vi "TSCAN_CANFD_Fold.vi"(10 "CANFD_Buffer输入":T1(array[cluster]), 11 "Fold Data":bool) -> (2 "CANFD_Buffer输出":T1(array[cluster]))   [LabVIEW 2014]
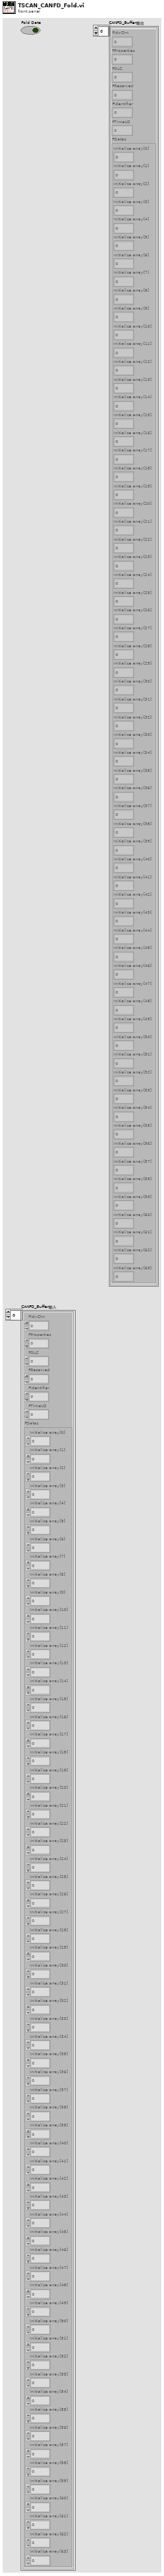
[diagram p1: front panel]
types:
  T1 = cluster{"FIdxChn":u8, "FProperties":u8, "FDLC":u8, "FReserved":u8, "FIdentifier":i32, "FTimeUS":u64, "FDatas":cluster{"Initialize array[0]":u8, "Initialize array[1]":u8, "Initialize array[2]":u8, "Initialize array[3]":u8, "Initialize array[4]":u8, "Initialize array[5]":u8, "Initialize array[6]":u8, "Initialize array[7]":u8, "Initialize array[8]":u8, "Initialize array[9]":u8, "Initialize array[10]":u8, "Initialize array[11]":u8, "Initialize array[12]":u8, "Initialize array[13]":u8, "Initialize array[14]":u8, "Initialize array[15]":u8, "Initialize array[16]":u8, "Initialize array[17]":u8, "Initialize array[18]":u8, "Initialize array[19]":u8, "Initialize array[20]":u8, "Initialize array[21]":u8, "Initialize array[22]":u8, "Initialize array[23]":u8, "Initialize array[24]":u8, "Initialize array[25]":u8, "Initialize array[26]":u8, "Initialize array[27]":u8, "Initialize array[28]":u8, "Initialize array[29]":u8, "Initialize array[30]":u8, "Initialize array[31]":u8, "Initialize array[32]":u8, "Initialize array[33]":u8, "Initialize array[34]":u8, "Initialize array[35]":u8, "Initialize array[36]":u8, "Initialize array[37]":u8, "Initialize array[38]":u8, "Initialize array[39]":u8, "Initialize array[40]":u8, "Initialize array[41]":u8, "Initialize array[42]":u8, "Initialize array[43]":u8, "Initialize array[44]":u8, "Initialize array[45]":u8, "Initialize array[46]":u8, "Initialize array[47]":u8, "Initialize array[48]":u8, "Initialize array[49]":u8, "Initialize array[50]":u8, "Initialize array[51]":u8, "Initialize array[52]":u8, "Initialize array[53]":u8, "Initialize array[54]":u8, "Initialize array[55]":u8, "Initialize array[56]":u8, "Initialize array[57]":u8, "Initialize array[58]":u8, "Initialize array[59]":u8, "Initialize array[60]":u8, "Initialize array[61]":u8, "Initialize array[62]":u8, "Initialize array[63]":u8}}[]
  T2 = cluster{"FIdxChn":u8, "FProperties":u8, "FDLC":u8, "FReserved":u8, "FIdentifier":i32, "FTimeUS":u64, "FDatas":cluster{"Initialize array[0]":u8, "Initialize array[1]":u8, "Initialize array[2]":u8, "Initialize array[3]":u8, "Initialize array[4]":u8, "Initialize array[5]":u8, "Initialize array[6]":u8, "Initialize array[7]":u8, "Initialize array[8]":u8, "Initialize array[9]":u8, "Initialize array[10]":u8, "Initialize array[11]":u8, "Initialize array[12]":u8, "Initialize array[13]":u8, "Initialize array[14]":u8, "Initialize array[15]":u8, "Initialize array[16]":u8, "Initialize array[17]":u8, "Initialize array[18]":u8, "Initialize array[19]":u8, "Initialize array[20]":u8, "Initialize array[21]":u8, "Initialize array[22]":u8, "Initialize array[23]":u8, "Initialize array[24]":u8, "Initialize array[25]":u8, "Initialize array[26]":u8, "Initialize array[27]":u8, "Initialize array[28]":u8, "Initialize array[29]":u8, "Initialize array[30]":u8, "Initialize array[31]":u8, "Initialize array[32]":u8, "Initialize array[33]":u8, "Initialize array[34]":u8, "Initialize array[35]":u8, "Initialize array[36]":u8, "Initialize array[37]":u8, "Initialize array[38]":u8, "Initialize array[39]":u8, "Initialize array[40]":u8, "Initialize array[41]":u8, "Initialize array[42]":u8, "Initialize array[43]":u8, "Initialize array[44]":u8, "Initialize array[45]":u8, "Initialize array[46]":u8, "Initialize array[47]":u8, "Initialize array[48]":u8, "Initialize array[49]":u8, "Initialize array[50]":u8, "Initialize array[51]":u8, "Initialize array[52]":u8, "Initialize array[53]":u8, "Initialize array[54]":u8, "Initialize array[55]":u8, "Initialize array[56]":u8, "Initialize array[57]":u8, "Initialize array[58]":u8, "Initialize array[59]":u8, "Initialize array[60]":u8, "Initialize array[61]":u8, "Initialize array[62]":u8, "Initialize array[63]":u8}}
  T3 = cluster{"FIdentifier":i32, "簇":cluster{"FIdxChn":u8, "FProperties":u8, "FDLC":u8, "FReserved":u8, "FIdentifier":i32, "FTimeUS":u64, "FDatas":cluster{"Initialize array[0]":u8, "Initialize array[1]":u8, "Initialize array[2]":u8, "Initialize array[3]":u8, "Initialize array[4]":u8, "Initialize array[5]":u8, "Initialize array[6]":u8, "Initialize array[7]":u8, "Initialize array[8]":u8, "Initialize array[9]":u8, "Initialize array[10]":u8, "Initialize array[11]":u8, "Initialize array[12]":u8, "Initialize array[13]":u8, "Initialize array[14]":u8, "Initialize array[15]":u8, "Initialize array[16]":u8, "Initialize array[17]":u8, "Initialize array[18]":u8, "Initialize array[19]":u8, "Initialize array[20]":u8, "Initialize array[21]":u8, "Initialize array[22]":u8, "Initialize array[23]":u8, "Initialize array[24]":u8, "Initialize array[25]":u8, "Initialize array[26]":u8, "Initialize array[27]":u8, "Initialize array[28]":u8, "Initialize array[29]":u8, "Initialize array[30]":u8, "Initialize array[31]":u8, "Initialize array[32]":u8, "Initialize array[33]":u8, "Initialize array[34]":u8, "Initialize array[35]":u8, "Initialize array[36]":u8, "Initialize array[37]":u8, "Initialize array[38]":u8, "Initialize array[39]":u8, "Initialize array[40]":u8, "Initialize array[41]":u8, "Initialize array[42]":u8, "Initialize array[43]":u8, "Initialize array[44]":u8, "Initialize array[45]":u8, "Initialize array[46]":u8, "Initialize array[47]":u8, "Initialize array[48]":u8, "Initialize array[49]":u8, "Initialize array[50]":u8, "Initialize array[51]":u8, "Initialize array[52]":u8, "Initialize array[53]":u8, "Initialize array[54]":u8, "Initialize array[55]":u8, "Initialize array[56]":u8, "Initialize array[57]":u8, "Initialize array[58]":u8, "Initialize array[59]":u8, "Initialize array[60]":u8, "Initialize array[61]":u8, "Initialize array[62]":u8, "Initialize array[63]":u8}}}
  T4 = cluster{"FIdentifier":i32, "簇":cluster{"FIdxChn":u8, "FProperties":u8, "FDLC":u8, "FReserved":u8, "FIdentifier":i32, "FTimeUS":u64, "FDatas":cluster{"Initialize array[0]":u8, "Initialize array[1]":u8, "Initialize array[2]":u8, "Initialize array[3]":u8, "Initialize array[4]":u8, "Initialize array[5]":u8, "Initialize array[6]":u8, "Initialize array[7]":u8, "Initialize array[8]":u8, "Initialize array[9]":u8, "Initialize array[10]":u8, "Initialize array[11]":u8, "Initialize array[12]":u8, "Initialize array[13]":u8, "Initialize array[14]":u8, "Initialize array[15]":u8, "Initialize array[16]":u8, "Initialize array[17]":u8, "Initialize array[18]":u8, "Initialize array[19]":u8, "Initialize array[20]":u8, "Initialize array[21]":u8, "Initialize array[22]":u8, "Initialize array[23]":u8, "Initialize array[24]":u8, "Initialize array[25]":u8, "Initialize array[26]":u8, "Initialize array[27]":u8, "Initialize array[28]":u8, "Initialize array[29]":u8, "Initialize array[30]":u8, "Initialize array[31]":u8, "Initialize array[32]":u8, "Initialize array[33]":u8, "Initialize array[34]":u8, "Initialize array[35]":u8, "Initialize array[36]":u8, "Initialize array[37]":u8, "Initialize array[38]":u8, "Initialize array[39]":u8, "Initialize array[40]":u8, "Initialize array[41]":u8, "Initialize array[42]":u8, "Initialize array[43]":u8, "Initialize array[44]":u8, "Initialize array[45]":u8, "Initialize array[46]":u8, "Initialize array[47]":u8, "Initialize array[48]":u8, "Initialize array[49]":u8, "Initialize array[50]":u8, "Initialize array[51]":u8, "Initialize array[52]":u8, "Initialize array[53]":u8, "Initialize array[54]":u8, "Initialize array[55]":u8, "Initialize array[56]":u8, "Initialize array[57]":u8, "Initialize array[58]":u8, "Initialize array[59]":u8, "Initialize array[60]":u8, "Initialize array[61]":u8, "Initialize array[62]":u8, "Initialize array[63]":u8}}}[]
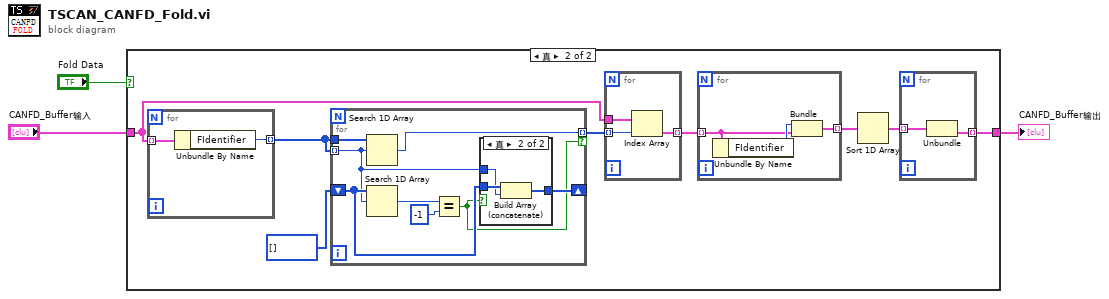
[diagram p0: block diagram]
diagram:
  n1 = case shown="真" "Fold Data" {
    tunnel: [w4 w11] -> w3
    tunnel: "CANFD_Buffer输入" -> [w4 w5]
    frame False {
    }
    frame True {
      n2 = for {
        tunnel: w5 -> [w29] mode=indexing
        tunnel: [w28] -> w8 mode=indexing
        n3 = Unbundle By Name(w29) -> ("FIdentifier"=w28:i32)
      }
      n4 = for {
        tunnel: w8 -> [w18] mode=indexing
        shift-right: [w23] -> _
        shift-left: u32[] [] -> [w22]
        tunnel: [w17] -> w6 mode=indexing if=w16
        tunnel: w8 -> [w19]
        n5 = Search 1D Array(1D array=w19, element=w18) -> (index of element=w17:i32)  [unwired: 1 in]
        n6 = Search 1D Array(1D array=w22, element=w18) -> (index of element=w20:i32)  [unwired: 1 in]
        n7 = Equal?(x=w20, y=-1) -> (x = y?=w16:bool)
        n8 = case shown="真" w16 {
          tunnel: [w24 w25] -> w23
          tunnel: w22 -> [w24 w27]
          tunnel: w18 -> [_ w26]
          frame False {
          }
          frame True {
            n9 = Build Array (concatenate)(w27, w26) -> (w25:u32[])
          }
        }
      }
      n10 = for {
        tunnel: w5 -> [w15]
        tunnel: w6 -> [w14] mode=indexing
        tunnel: [w13] -> w12 mode=indexing
        n11 = Index Array(array=w15, index=w14) -> (element=w13:T2)
      }
      n12 = for {
        tunnel: w12 -> [w33] mode=indexing
        tunnel: [w32] -> w10 mode=indexing
        n13 = Unbundle By Name(w33) -> ("FIdentifier"=w34:i32)
        n14 = Bundle("FIdentifier"=w34, "簇"=w33) -> (w32:T3)  [unwired: 1 in]
      }
      n15 = Sort 1D Array(array=w10) -> (sorted array=w9:T4)
      n16 = for {
        tunnel: w9 -> [w31] mode=indexing
        tunnel: [w30] -> w11 mode=indexing
        n17 = Unbundle(w31) -> ("簇"=w30:T2)  [unwired: 1 out]
      }
    }
  }
  "CANFD_Buffer输出" <- w3
